vi "min_max_from_span_center.vi"(3 "No Points":i32, 4 "Mid Point":dbl, 5 "Span":dbl) -> (0 "Step":dbl, 1 "Start":dbl, 2 "End":dbl)   [LabVIEW 2013]
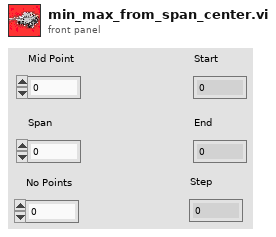
[diagram p1: front panel]
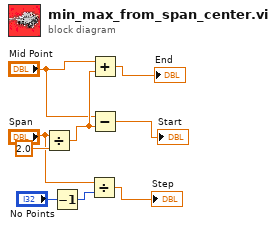
[diagram p0: block diagram]
diagram:
  n1 = Divide(x="Span", y=2.0) -> (x/y=w7:dbl)
  n2 = Decrement(x="No Points") -> (x-1=w3:i32)
  n3 = Divide(x="Span", y=w3) -> (x/y=→"Step":dbl)
  n4 = Add(x="Mid Point", y=w7) -> (x+y=→"End":dbl)
  n5 = Subtract(x="Mid Point", y=w7) -> (x-y=→"Start":dbl)
